vi "test_Enable Periodic Message Channel.vi"(8 "error in (no error)":errorcluster, 11 "TestCase in":refnum<class "Instrument Addon Common System Tests.lvclass">) -> (0 "error out":errorcluster, 3 "TestCase out":refnum<class "Instrument Addon Common System Tests.lvclass">)   [LabVIEW 2019, in "Instrument Addon Common System Tests.lvclass"]
uses:
  Instrument Addon Common System Tests.lvclass
  <vilib>/addons/_JKI Toolkits/VI Tester/TestCase.llb/TestCase.lvclass
  <vilib>/NI VeriStand/Execution/Workspace/NI_VS Workspace ExecutionAPI.lvlib
  <vilib>/NI VeriStand/Execution/Workspace/NI VeriStand - Get Multiple Channel Values.vi
  <vilib>/NI VeriStand/Execution/Workspace/NI VeriStand - Set Single Channel Value.vi
  C:/Users/nitest/Desktop/Git 2019/niveristand-custom-device-testing-tools/VeriStandTestCase/VeriStandTestCase.lvclass
  C:/Program Files (x86)/National Instruments/LabVIEW 2019/vi.lib/addons/_JKI Toolkits/VI Tester/TestCase.llb/TestCase.lvclass
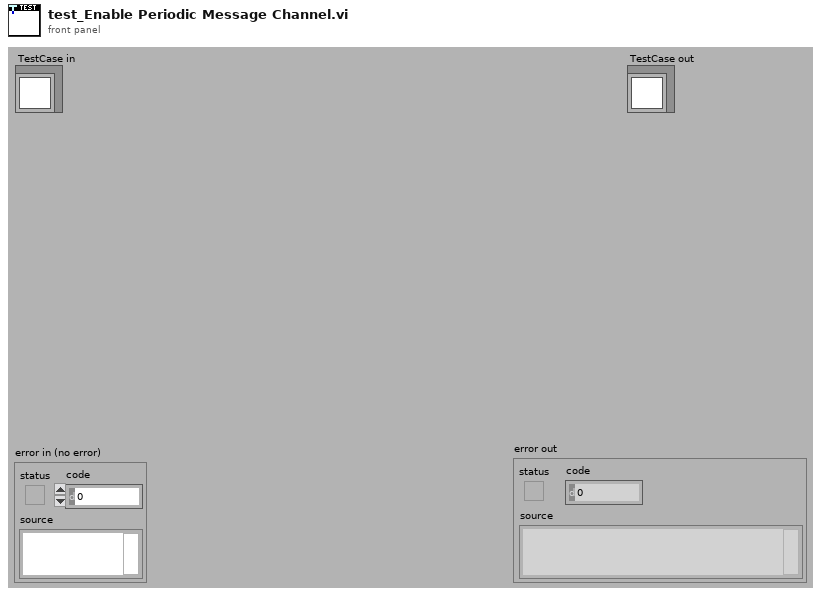
[diagram p1: front panel]
types:
  T1 = typedef "NI_VS Workspace ExecutionAPI.lvlib/WorkspaceAPI.ctl" = refnum<k24>
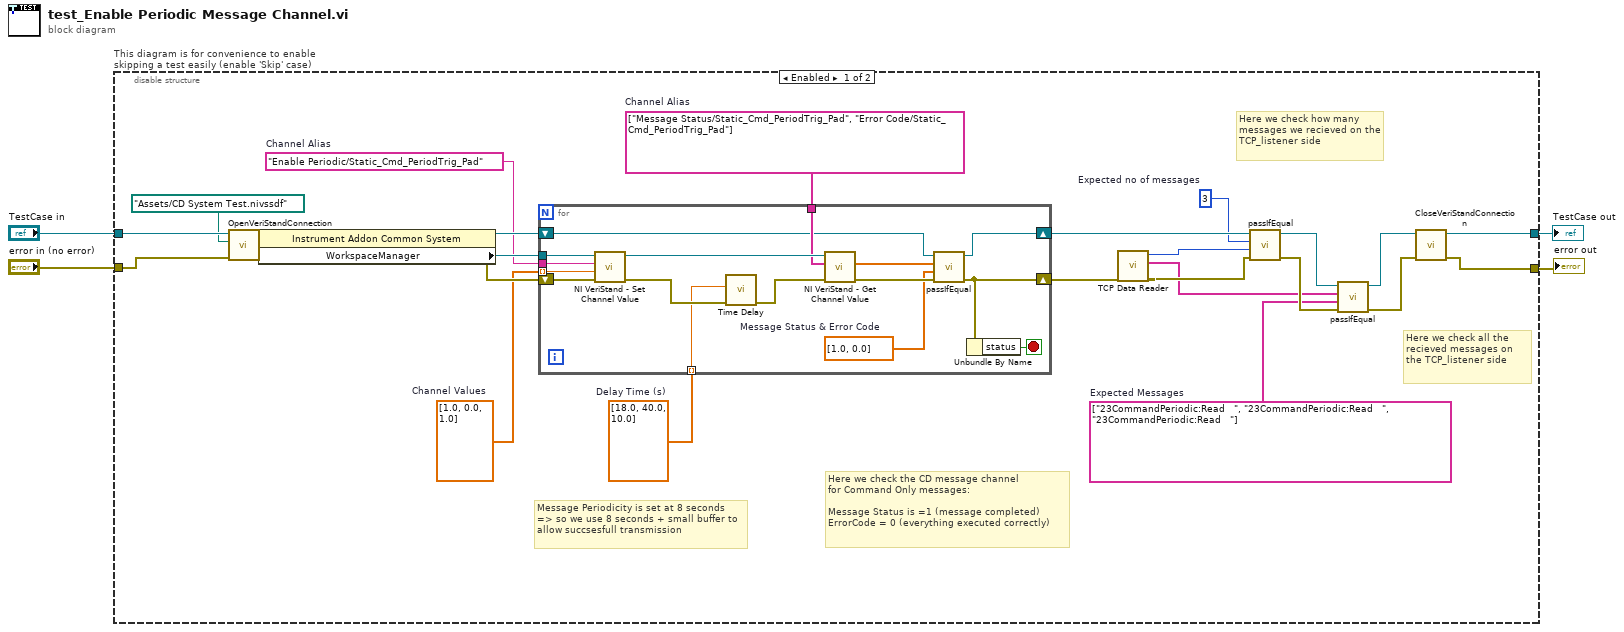
[diagram p0: block diagram]
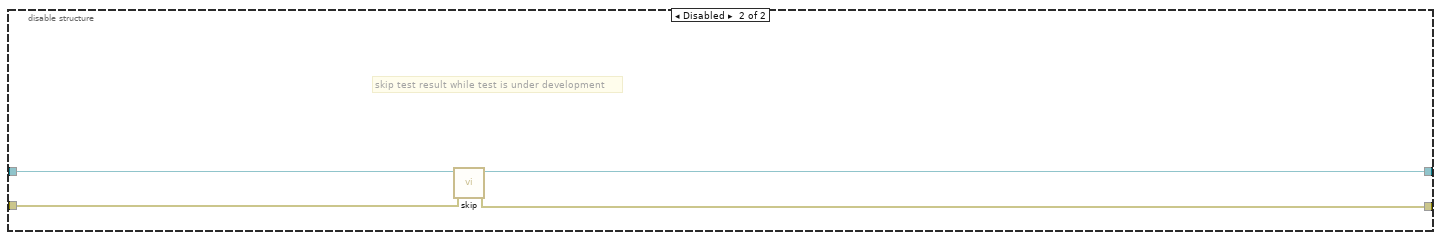
[diagram p2: hidden frame]
diagram:
  n1 = disable-structure "This diagram is for convenience to enable skipping a test easily (enable 'Skip' case)" shown="Enabled" {
    disable-tunnel: "TestCase in" -> [w27 w49]
    disable-tunnel: [w28 w47] -> w1
    disable-tunnel: [w29 w48] -> w3
    disable-tunnel: "error in (no error)" -> [w25 w46]
    frame Enabled {
      w5 = "Enable Periodic/Static_Cmd_PeriodTrig_Pad"  # Channel Alias
      w6 = dbl[] [18.0, 40.0, 10.0]  # Delay Time (s)
      w12 = string[] ["23CommandPeriodic:Read   ", "23CommandPeriodic:Read   ", "23CommandPeriodic:Read   "]  # Expected Messages
      w14 = string[] ["Message Status/Static_Cmd_PeriodTrig_Pad", "Error Code/Static_Cmd_PeriodTrig_Pad"]  # Channel Alias
      w11 = 3  # Expected no of messages
      w20 = dbl[] [1.0, 0.0, 1.0]  # Channel Values
      # "Message Periodicity is set at 8 seconds\n=> so we use 8 seconds + small buffer to allow succsesfull transmission"
      # "Here we check all the recieved messages on the TCP_listener side"
      # "Here we check how many messages we recieved on the TCP_listener side"
      # "Here we check the CD message channel\nfor Command Only messages:\n\nMessage Status is =1 (message completed)\nErrorCode = 0 (everything executed correctly)"
      n2 = call-dynamic "OpenVeriStandConnection.vi"("error in (no error)"=w25, "System Definition File"=path "Assets/CD System Test.nivssdf", "VeriStand Test Case in"=w27) -> ("error out"=w24:errorcluster, "VeriStand Test Case out"=w26:refnum<class "Instrument Addon Common System Tests.lvclass">)  [unwired: 6 in, 1 out]
      n3 = property class="Instrument Addon Common System "(reference=w26, error in=w24) -> (reference out=w19:refnum<class "Instrument Addon Common System Tests.lvclass">, error out=w21:errorcluster, "WorkspaceManager"=w22:T1)
      n4 = for {
        tunnel: w22 -> [w45]
        tunnel: w5 -> [w43]
        tunnel: w20 -> [w42] mode=indexing
        shift-right: [w32] -> w10
        shift-left: w21 -> [w44]
        tunnel: w14 -> [w40]
        shift-right: [w36] -> w13
        shift-left: w19 -> [w37]
        tunnel: w6 -> [w30] mode=indexing
        stop <- w31 stop-if-true
        w33 = dbl[] [1.0, 0.0]  # Message Status & Error Code
        n5 = call-poly <vilib>:"NI VeriStand - Set Channel Value.vi"("error in (no error)"=w44, "Value"=w42, "Channel"=w43, "WorkspaceManager in"=w45) -> ("error out"=w39:errorcluster, "WorkspaceManager out"=w41:T1)  [unwired: 6 in]
        n6 = call "Time Delay"("error in (no error)"=w39, "Delay Time (s)"=w30) -> ("error out"=w38:errorcluster)  [unwired: 9 in]
        n7 = call-poly <vilib>:"NI VeriStand - Get Channel Value.vi"("error in (no error)"=w38, "Channels"=w40, "WorkspaceManager in"=w41) -> ("error out"=w35:errorcluster, "Values"=w34:dbl[])  [unwired: 6 in, 1 out]
        n8 = call-dynamic "passIfEqual.vi"("error in (no error)"=w35, "y"=w33, "x"=w34, "TestCase in"=w37) -> ("error out"=w32:errorcluster, "TestCase out"=w36:refnum<class "Instrument Addon Common System Tests.lvclass">)  [unwired: 6 in]
        n9 = Unbundle By Name(w32) -> ("status"=w31:bool)
      }
      n10 = call "TCP Data Reader.vi"("error in (no error)"=w10) -> ("error out"=w8:errorcluster, "Recieved Messages"=w7:string[], "No of messages"=w9:i32)  [unwired: 8 in]
      n11 = call-dynamic "passIfEqual.vi"("error in (no error)"=w8, "y"=w9, "x"=w11, "TestCase in"=w13) -> ("error out"=w16:errorcluster, "TestCase out"=w18:refnum<class "Instrument Addon Common System Tests.lvclass">)  [unwired: 6 in]
      n12 = call-dynamic "passIfEqual.vi"("error in (no error)"=w16, "y"=w12, "x"=w7, "TestCase in"=w18) -> ("error out"=w15:errorcluster, "TestCase out"=w17:refnum<class "Instrument Addon Common System Tests.lvclass">)  [unwired: 6 in]
      n13 = call-dynamic "CloseVeriStandConnection.vi"("error in (no error)"=w15, "VeriStand Test Case in"=w17) -> ("error out"=w29:errorcluster, "VeriStand Test Case out"=w28:refnum<class "Instrument Addon Common System Tests.lvclass">)  [unwired: 8 in]
    }
    frame Disabled {
      # "skip test result while test is under development"
      n14 = call <vilib>:"skip.vi"("error in (no error)"=w46, "TestCase in"=w49) -> ("error out"=w48:errorcluster, "TestCase out"=w47:refnum<class "Instrument Addon Common System Tests.lvclass">)  [unwired: 8 in]
    }
  }
  "error out" <- w3
  "TestCase out" <- w1
